vi "Zonal Stats to CVT.vi"(8 "error in (no error)":errorcluster, 10 "StatisticsData":T2, 11 "Pamameter":T1) -> (0 "error out":errorcluster)   [LabVIEW 2020]
uses:
  StatisticsData.ctl
  CompressAndUpdate(Numeric).vi
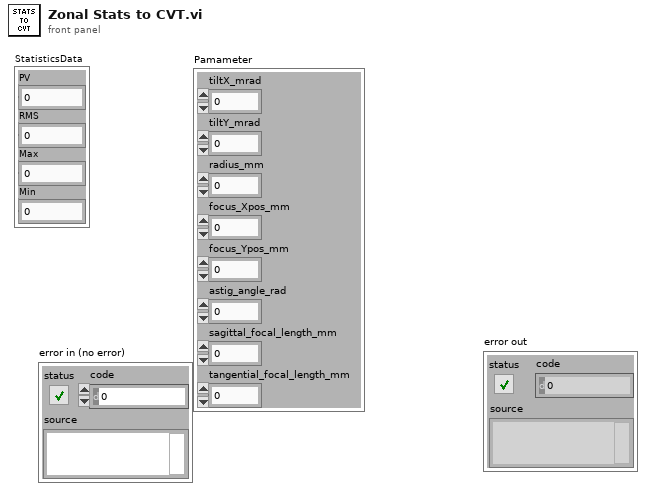
[diagram p1: front panel]
types:
  T1 = cluster{"tiltX_mrad":sgl, "tiltY_mrad":dbl, "radius_mm":sgl, "focus_Xpos_mm":sgl, "focus_Ypos_mm":sgl, "astig_angle_rad":sgl, "sagittal_focal_length_mm":sgl, "tangential_focal_length_mm":sgl}
  T2 = typedef "StatisticsData.ctl" = cluster{"PV":sgl, "RMS":dbl, "Max":sgl, "Min":sgl}
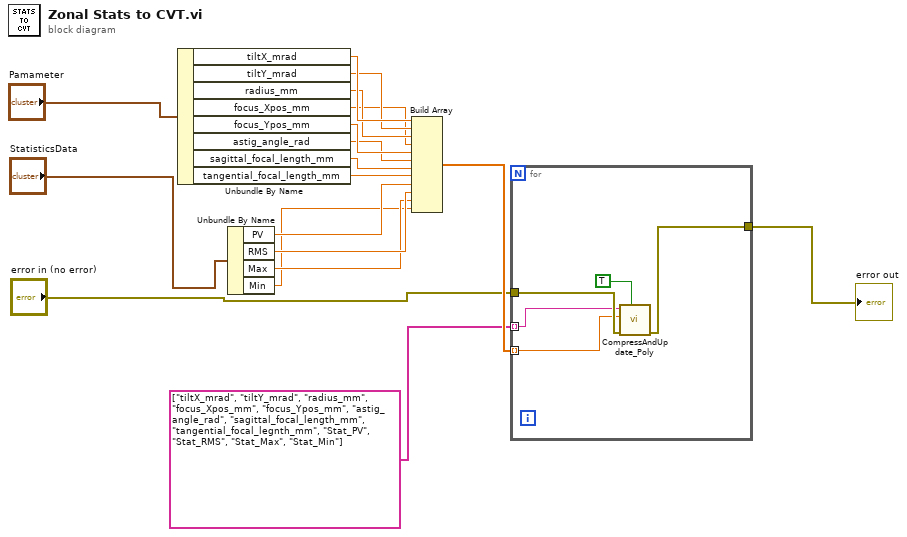
[diagram p0: block diagram]
diagram:
  n1 = Unbundle By Name("Pamameter") -> ("tiltX_mrad"=w18:sgl, "tiltY_mrad"=w17:dbl, "radius_mm"=w16:sgl, "focus_Xpos_mm"=w15:sgl, "focus_Ypos_mm"=w14:sgl, "astig_angle_rad"=w13:sgl, "sagittal_focal_length_mm"=w12:sgl, "tangential_focal_length_mm"=w11:sgl)
  n2 = Unbundle By Name("StatisticsData") -> ("PV"=w10:sgl, "RMS"=w9:dbl, "Max"=w8:sgl, "Min"=w7:sgl)
  n3 = Build Array(w18, w17, w16, w15, w14, w13, w12, w11, w10, w9, w8, w7) -> (w4:dbl[])
  n4 = for {
    tunnel: w4 -> [w21] mode=indexing
    tunnel: string[] ["tiltX_mrad", "tiltY_mrad", "radius_mm", "focus_Xpos_mm", "focus_Ypos_mm", "astig_angle_rad", "sagittal_focal_length_mm", "tangential_focal_legnth_mm", "Stat_PV", "Stat_RMS", "Stat_Max", "Stat_Min"] -> [w20] mode=indexing
    tunnel: "error in (no error)" -> [w23]
    tunnel: [w22] -> w1
    n5 = call-poly "CompressAndUpdate_Poly.vi"("force CVT update (false)"=TRUE, "error in"=w23, "Numeric"=w21, "command or variable name"=w20) -> ("error out"=w22:errorcluster)  [unwired: 7 in]
  }
  "error out" <- w1
